vi "mod_FM CE Demodulation (block processing).vi"(5 "reset?":bool, 6 "carrier correction?":bool, 7 "weighting window":T1(ring)=enum."Hanning", 8 "kf":dbl format="%.2p", 9 "remove transient on reset?":bool, 10 "fs":dbl format="%.2p", 11 "x":cdb[](array[numeric]) format="%.2f") -> (0 "filter length":i32, 1 "carrier frequency":dbl format="%.2f", 3 "FM demod":dbl[](array[numeric]) format="%.2f", 4 "# transient samples truncated":i32)   [LabVIEW 2020, in "niAMT.lvlib"]
doc: "This VI performs FM demodulation for incoming analog I-Q signal. Basically the input signal is the base band I-Q signal with possible some carrier offset. If the carrier correction boolean is on, this VI will perform weighted linear fit to estimate the carrier frequency. The weighting function can be chosen from a variety of window functions. The estimated value will be returned as carrier frequency in hertz. If the boolean is off, this value will be set to zero.\nInternally, this VI performs PM demodulation first, FM signal is acquired via dirivative of PM signal."
uses:
  <vilib>/addons/Modulation/niAMT.lvlib
  <vilib>/addons/Modulation/Analog/controls/mod_FM demod state.ctl
  nilvamt.dll
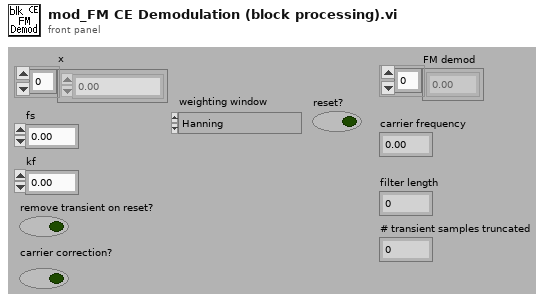
[diagram p1: front panel]
types:
  T1 = enum16{"None ", "Hanning", "Hamming", "Blackman-Harris", "Exact Blackman", "Blackman", "Flat Top", "4 Term B-Harris ", "7 Term B-Harris", "Low Sidelobe"}
  T2 = typedef "niAMT.lvlib/mod_FM demod state.ctl" = cluster{"lastPhase":dbl, "lp2":dbl, "lp2":dbl, "scalingFactor":dbl, "sum":dbl, "n":dbl}
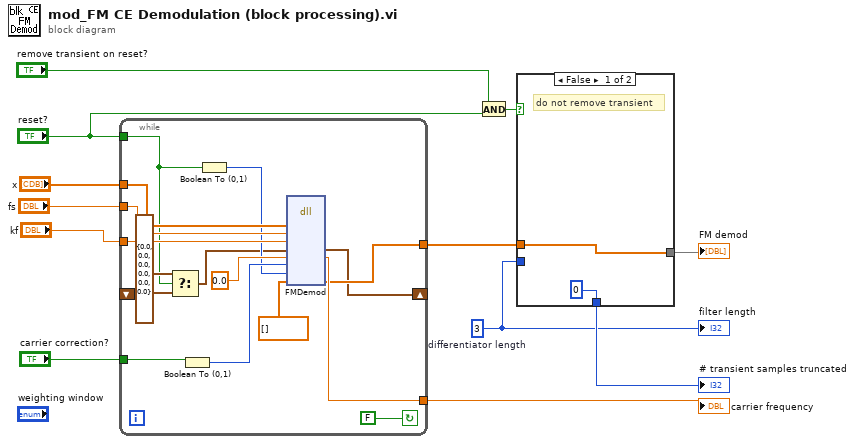
[diagram p0: block diagram]
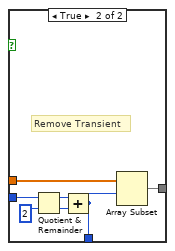
[diagram p2: hidden frame]
diagram:
  w1 = 3  # differentiator length
  n1 = while {
    tunnel: "x" -> [w28]
    tunnel: "fs" -> [w27]
    tunnel: "kf" -> [w26]
    tunnel: [w25] -> w5
    tunnel: "carrier correction?" -> [w23]
    tunnel: "reset?" -> [w15]
    tunnel: [w19] -> w2
    shift-right: [w13] -> _
    shift-left: _ -> [w16]
    stop <- FALSE continue-if-true
    n2 = Select(t=T2 {"lastPhase"=0.0, "lp2"=0.0, "lp2"=0.0, "scalingFactor"=0.0, "sum"=0.0, "n"=0.0} ("FM demod state"), s=w15, f=w16) -> (s? t:f=w14:T2)
    n3 = Boolean To (0,1)(Boolean=w23) -> (0, 1=w22:i16)
    n4 = Boolean To (0,1)(Boolean=w15) -> (0, 1=w21:i16)
    n5 = dll-call lib="nilvamt.*" fn="FMDemod"("x"=w28, "fs"=w27, "kf"=w26, "state"=w14, "freqOffset"=0.0, "carrierOffsetCorrection"=w22, "reset"=w21, "m"=dbl[] []) -> ("state"=w13:T2, "freqOffset"=w25:dbl, "m"=w19:dbl[])  [unwired: 4 in, 7 out]
  }
  "carrier frequency" <- w5
  n6 = And(x="remove transient on reset?", y="reset?") -> (x .and. y?=w9:bool)
  n7 = case shown="False" w9 {
    tunnel: w2 -> [w30 w32]
    tunnel: [w30 w31] -> w11
    tunnel: w1 -> [_ w37]
    tunnel: [0 w33] -> w10
    frame False {
      # "do not remove transient"
    }
    frame True {
      # "Remove Transient"
      n8 = Quotient & Remainder(x=w37, y=2) -> (x-y*floor(x/y)=w34:i32, floor(x/y)=w35:i32)
      n9 = Add(x=w34, y=w35) -> (x+y=w33:i32)
      n10 = Array Subset(array=w32, index=w33) -> (w31:dbl[])  [unwired: 1 in]
    }
  }
  "FM demod" <- w11
  "# transient samples truncated" <- w10
  "filter length" <- w1
